vi "ReadExcel.vi"(8 "error in (no error)":errorcluster caption="错误输入（无错误）", 11 "Path":path=path "C:/Users/ct/Desktop/TestStep.xlsx") -> (0 "error out":errorcluster caption="错误输出", 3 "OutPut Data":string[][](array[string]))   [LabVIEW 2017]
uses:
  <vilib>/addons/_office/NI_ReportGenerationToolkit.lvlib
  <vilib>/addons/_office/excel.llb/Excel Get Data ([str]).vi
  <vilib>/Utility/NIReport.llb/Excel/NI_Excel.lvclass
  <vilib>/Utility/NIReport.llb/NI_report.lvclass
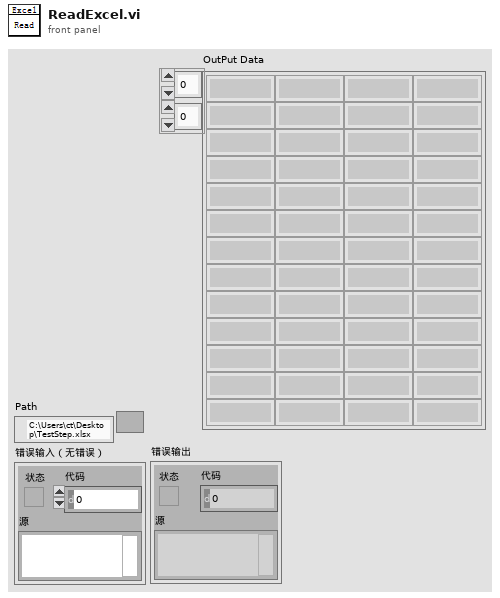
[diagram p1: front panel]
types:
  T1 = enum16{"Standard Report", "HTML", "Word", "Excel"}
  T2 = enum16{"maximized", "minimized", "normal", "no change"}
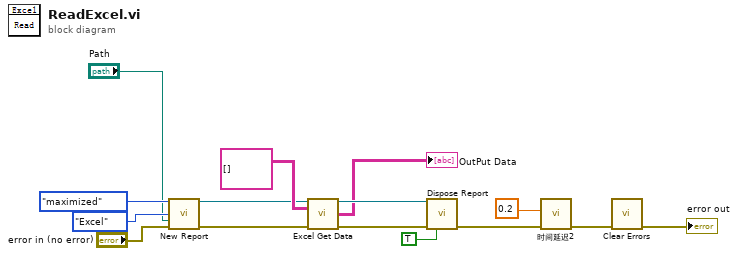
[diagram p0: block diagram]
diagram:
  n1 = call <vilib>:"New Report.vi"("window state (normal)"=T2."maximized", "report type"=T1."Excel", "template (empty)"="Path", "error in (no error)"="error in (no error)") -> ("report out"=w11:refnum<class "NI_report.lvclass">, "error out"=w10:errorcluster)  [unwired: 10 in]
  n2 = call-poly <vilib>:"Excel Get Data.vi"("report in"=w11, "data type"=string[][] [], "error in (no error)"=w10) -> ("report out"=w8:refnum<class "NI_report.lvclass">, "data"=→"OutPut Data":string[][], "error out"=w5:errorcluster)  [unwired: 10 in]
  n3 = call-dynamic "Dispose Report.vi"("report in"=w8, "error in (no error)"=w5, "close report? (T)"=TRUE) -> ("error out"=w3:errorcluster)  [unwired: 12 in]
  n4 = call "时间延迟2"("error in (no error)"=w3, "Delay Time (s)"=0.2) -> ("error out"=w2:errorcluster)  [unwired: 9 in]
  n5 = call <vilib>:"Clear Errors.vi"("error in (no error)"=w2) -> ("error out"=→"error out":errorcluster)  [unwired: 5 in, 1 out]
